vi "Sweep List.vi"() -> ()   [LabVIEW 2016]
panel:
  out "Sweep List":dbl[](array[numeric])
  out "Step Size (V)":dbl
  in  "Forward/Reverse":bool
  in  "Step Number":dbl
  in  "Start (V)":dbl
  in  "Stop (V)":dbl
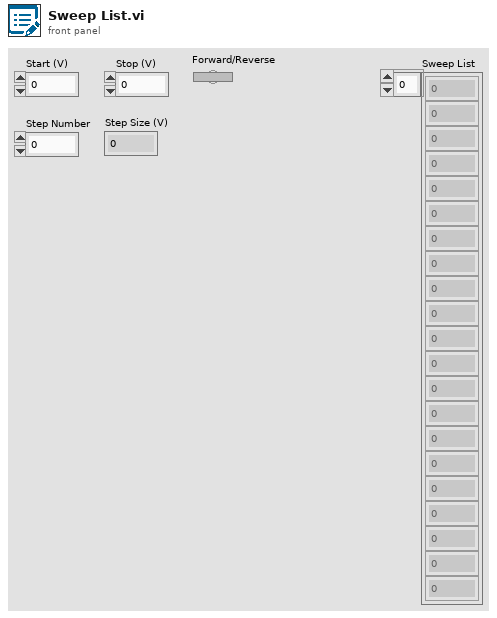
[diagram p1: front panel]
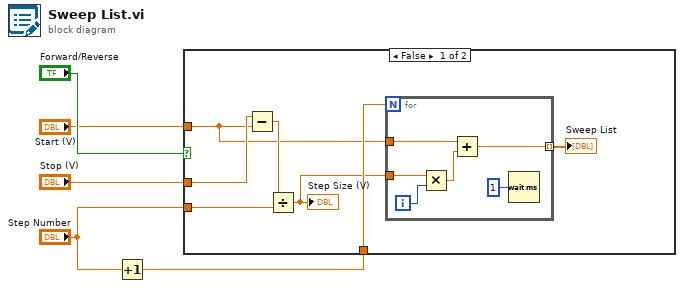
[diagram p0: block diagram]
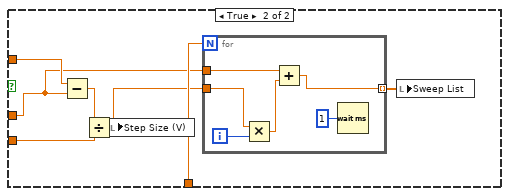
[diagram p2: hidden frame]
diagram:
  n1 = Increment(x="Step Number") -> (x+1=w2:dbl)
  n2 = case shown="False" "Forward/Reverse" {
    tunnel: "Stop (V)" -> [w12 w23]
    tunnel: "Start (V)" -> [w8 w25]
    tunnel: w2 -> [w11 w24]
    tunnel: "Step Number" -> [w9 w21]
    frame False {
      n3 = Subtract(x=w12, y=w8) -> (x-y=w10:dbl)
      n4 = Divide(x=w10, y=w9) -> (x/y=w7:dbl)
      "Step Size (V)" <- w7
      n5 = for {
        N: w11 -> [_]
        tunnel: w8 -> [w18]
        tunnel: w7 -> [w16]
        tunnel: [w14] -> w6 mode=indexing
        i -> [w17]
        n6 = Multiply(x=w16, y=w17) -> (x*y=w15:dbl)
        n7 = Add(x=w18, y=w15) -> (x+y=w14:dbl)
        n8 = Wait (ms)(milliseconds to wait=u32 1) -> ()  [unwired: 1 out]
      }
      "Sweep List" <- w6
    }
    frame True {
      n9 = Subtract(x=w25, y=w23) -> (x-y=w20:dbl)
      n10 = Divide(x=w20, y=w21) -> (x/y=w19:dbl)
      n11 = local write "Step Size (V)"(w19) -> ()
      n12 = for {
        N: w24 -> [_]
        tunnel: w19 -> [w30]
        tunnel: w23 -> [w28]
        tunnel: [w27] -> w22 mode=indexing
        i -> [w31]
        n13 = Multiply(x=w30, y=w31) -> (x*y=w29:dbl)
        n14 = Add(x=w28, y=w29) -> (x+y=w27:dbl)
        n15 = Wait (ms)(milliseconds to wait=u32 1) -> ()  [unwired: 1 out]
      }
      n16 = local write "Sweep List"(w22) -> ()
    }
  }
